vi "steering frame.vi"() -> ()   [LabVIEW 2011]
uses:
  <vilib>/robotics/Steering/Wheel/Wheel Parameters.ctl
  <vilib>/robotics/Steering/Wheel/Rotation Direction.ctl
  <vilib>/robotics/Steering/Fixed Wheel/Create Fixed Wheel.vi
  <vilib>/robotics/Steering/Differential Steering Frame/Create Differential Steering Frame.vi
  <vilib>/robotics/Steering/Steering Frame/Apply Steering Frame Velocity to Motors.vi
  <vilib>/robotics/Steering/Wheel/NI_Robotics_Wheel.lvclass
  <vilib>/robotics/Steering/Fixed Wheel/NI_Robotics_Fixed Wheel.lvclass
  <vilib>/robotics/Steering/Steering Frame/NI_Robotics_Steering Frame.lvclass
  <vilib>/robotics/Actuation/Motor Communication/NI_Robotics_Motor Communication.lvclass
  <vilib>/robotics/Steering/Differential Steering Frame/NI_Robotics_Differential Steering Frame.lvclass
panel:
  in  "wheel parameters":T1={"wheel radius"=1.0, "gear ratio"=1.0, "forward rotation direction"=enum."Clockwise"}
  in  "error in (no error)":errorcluster
  in  "steering frame velocity":dbl[](array[numeric])=[0.0, 0.0, 0.0]
  in  "wheel separation":dbl
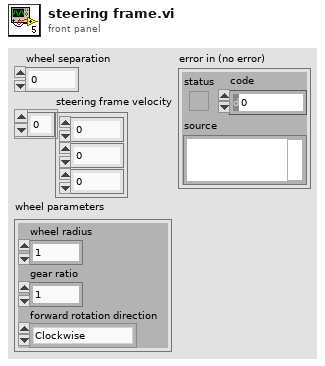
[diagram p1: front panel]
types:
  T1 = typedef "NI_Robotics_Wheel.lvclass/Wheel Parameters.ctl" = cluster{"wheel radius":dbl, "gear ratio":dbl, "forward rotation direction":T2}
  T2 = typedef "NI_Robotics_Wheel.lvclass/Rotation Direction.ctl" = enum16{"Clockwise", "Counterclockwise"}
  T3 = cluster{"fixed wheel out":refnum<class "NI_Robotics_Fixed Wheel.lvclass">, "fixed wheel out":refnum<class "NI_Robotics_Fixed Wheel.lvclass">}
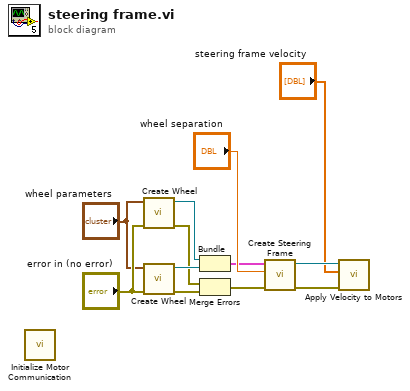
[diagram p0: block diagram]
diagram:
  n1 = call <vilib>:"Initialize Motor Communication.vi"() -> ()  [unwired: 10 in, 2 out]
  n2 = call-poly <vilib>:"Create Wheel.vi"("error in (no error)"="error in (no error)", "wheel parameters"="wheel parameters") -> ("error out"=w5:errorcluster, "fixed wheel out"=w11:refnum<class "NI_Robotics_Fixed Wheel.lvclass">)  [unwired: 8 in]
  n3 = call-poly <vilib>:"Create Wheel.vi"("error in (no error)"="error in (no error)", "wheel parameters"="wheel parameters") -> ("error out"=w4:errorcluster, "fixed wheel out"=w10:refnum<class "NI_Robotics_Fixed Wheel.lvclass">)  [unwired: 8 in]
  n4 = Bundle("fixed wheel out"=w11, "fixed wheel out"=w10) -> (w9:T3)  [unwired: 1 in]
  n5 = Merge Errors(w5, w4) -> (w3:errorcluster)
  n6 = call-poly <vilib>:"Create Steering Frame.vi"("error in (no error)"=w3, "wheel separation"="wheel separation", "wheels"=w9) -> ("error out"=w6:errorcluster, "differential steering frame out"=w8:refnum<class "NI_Robotics_Differential Steering Frame.lvclass">)  [unwired: 7 in]
  n7 = call-poly <vilib>:"Apply Velocity to Motors.vi"("error in (no error)"=w6, "steering frame velocity"="steering frame velocity", "steering frame in"=w8) -> ()  [unwired: 4 in, 5 out]
